vi "currentMax.vi"(8 "error in (no error)":errorcluster, 11 "VISA Refnum in":refnum<visa-resource-name>) -> (0 "error out":errorcluster, 2 "stringCurrentMax":string, 3 "numberCurrentMax":dbl)   [LabVIEW 2018]
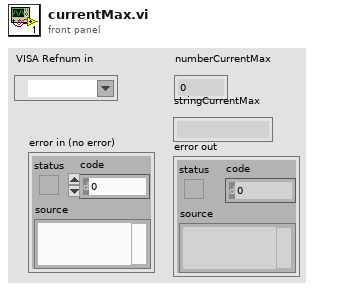
[diagram p1: front panel]
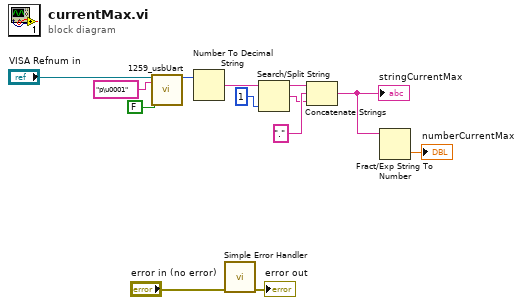
[diagram p0: block diagram]
diagram:
  n1 = call "1259_usbUart.vi"("VISA resource name"="VISA Refnum in", "write buffer"="p\u0001", "sdFeature"=FALSE) -> ("number[0]"=w11:u32)  [unwired: 1 in, 15 out]
  n2 = Number To Decimal String(number=w11) -> (decimal integer string=w12:string)  [unwired: 1 in]
  n3 = call <vilib>:"Simple Error Handler.vi"("error in (no error)"="error in (no error)") -> ("error out"=→"error out":errorcluster)  [unwired: 4 in, 4 out]
  n4 = Search/Split String(string=w12, offset (0)=1) -> (substring before match=w5:string, match + rest of string=w4:string)  [unwired: 1 in, 1 out]
  n5 = Concatenate Strings(w5, "." ("string"), w4) -> (w8:string)
  "stringCurrentMax" <- w8
  n6 = Fract/Exp String To Number(string=w8) -> (number=→"numberCurrentMax":dbl)  [unwired: 3 in, 1 out]
